vi "Smart Home Project.vi"() -> ()   [LabVIEW 2014]
doc: "This example demonstrates how to read one channel of digital input from a LINX device."
uses:
  <vilib>/MakerHub/LINX/Public/Peripherals/Digital/Digital Read 1 Chan.vi
  <vilib>/MakerHub/LINX/Public/Peripherals/Digital/Digital Write 1 Chan.vi
  <vilib>/MakerHub/LINX/Public/Peripherals/Analog/Analog Read 1 Chan.vi
  <vilib>/MakerHub/LINX/Public/Peripherals/PWM/PWM Set Duty Cycle 1 Chan.vi
  <vilib>/MakerHub/LINX/Public/Peripherals/Digital/Digital Read N Chans.vi
  <vilib>/MakerHub/LINX/Public/Peripherals/Digital/Digital Write N Chans.vi
  <vilib>/MakerHub/LINX/Public/Peripherals/Analog/Analog Read N Chans.vi
  <vilib>/MakerHub/LINX/Private/Local IO/LinxDigitalRead.vi
  <vilib>/MakerHub/LINX/Public/Utilities/Check Channel.vi
  <vilib>/MakerHub/LINX/Private/Local IO/LinxDigitalWrite.vi
  <vilib>/MakerHub/LINX/Private/Local IO/LinxAnalogRead.vi
  <vilib>/MakerHub/LINX/Public/Utilities/Open Serial.vi
  <vilib>/MakerHub/LINX/Public/Sensors/Motion/Servo/Servo Open One Channel.vi
  <vilib>/MakerHub/LINX/Private/Utilties/Generate Error.vi
  <vilib>/MakerHub/LINX/Public/Peripherals/PWM/PWM Set Duty Cycle N Chans.vi
  <vilib>/MakerHub/LINX/Public/Sensors/Motion/Servo/Servo Set Pulse Width One Channel.vi
  <vilib>/MakerHub/LINX/Public/Sensors/Motion/Servo/Servo Close One Channel.vi
  <vilib>/MakerHub/LINX/LMH-LINX.lvlib
  <vilib>/MakerHub/LINX/Public/Sensors/Motion/Servo/Servo.lvlib
panel:
  out "LDR Value":dbl
  out "Temp":dbl(slide) scale=0.0..50.0
  in  "Stop Button":bool
  out "TCR":bool
  out "Sound Sensor  Case":bool
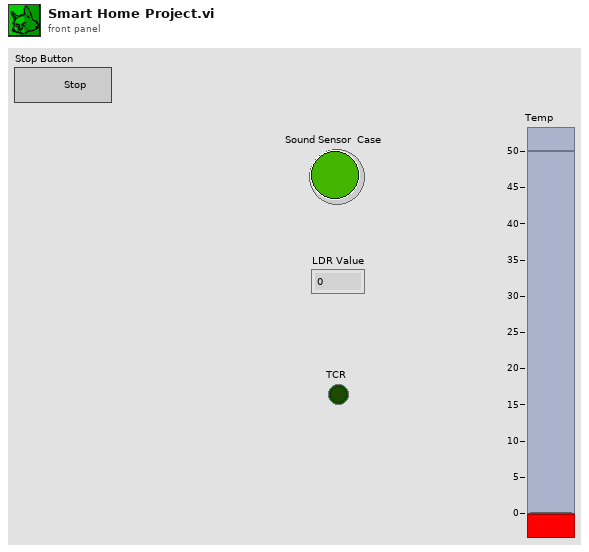
[diagram p1: front panel]
types:
  T1 = typedef "LMH-LINX.lvlib/LINX Ref.ctl" = cluster{"IO":T2, "Interface":T3, "LINX Device Config":T4}
  T2 = typedef "LMH-LINX.lvlib/Platform.ctl" = enum16{"Remote", "Local"}
  T3 = typedef "LMH-LINX.lvlib/Interface.ctl" = enum16{"Serial", "TCP"}
  T4 = typedef "LMH-LINX.lvlib/Device.lvlib/LINX Device Config.ctl" = cluster{"Interface":T3, "COM Port":refnum<visa-resource-name>, "TCP Configuration":T5, "Device Family":u8, "Device ID":u8, "Device Name":string, "TCP Ref":refnum<k5>, "Channels":T6}
  T5 = typedef "LMH-LINX.lvlib/Device.lvlib/TCP Config.ctl" = cluster{"IP Address":string, "Port":u16}
  T6 = typedef "LMH-LINX.lvlib/Channels.ctl" = cluster{"DI":u8[], "DO":u8[], "AI":u8[], "AO":u8[], "PWM":u8[], "QE":u8[], "UART":u8[], "I2C 2":u8[], "SPI":u8[], "CAN":u8[], "Servo":u8[], "AI Ref (V)":dbl, "AI Resolution (Bits)":u8, "AO Ref (V)":dbl, "AO Resolution (Bits)":u8}
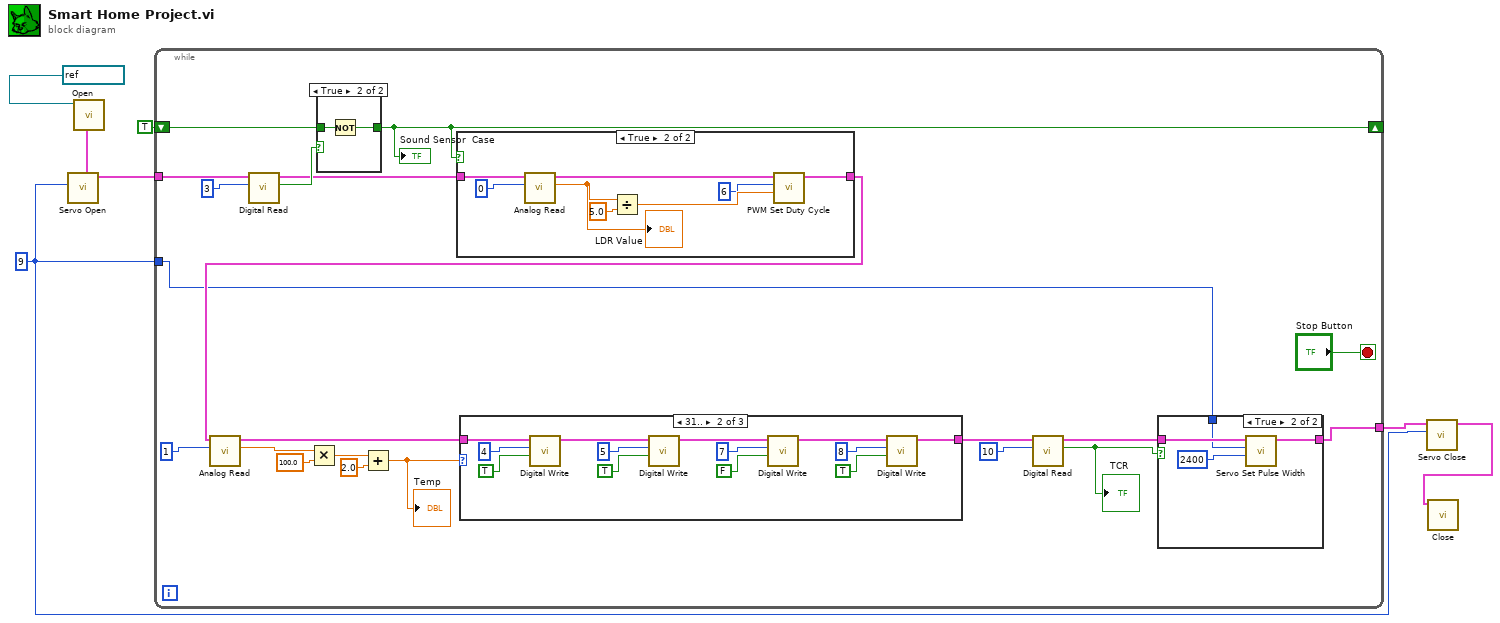
[diagram p0: block diagram]
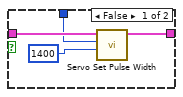
[diagram p2: hidden frame]
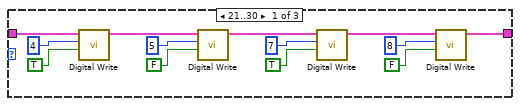
[diagram p3: hidden frame]
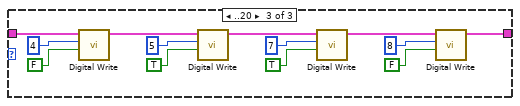
[diagram p4: hidden frame]
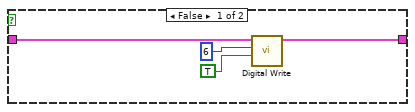
[diagram p5: hidden frame]
diagram:
  w1 = u8 9 ("Servo Channel")
  n1 = call-poly <vilib>:"Open.vi"("Serial Port"=refnum<visa-resource-name> "COM3") -> ("LINX Resource"=w4:T1)  [unwired: 8 in, 2 out]
  n2 = call-poly <vilib>:"Servo Open.vi"("Servo Channel"=w1, "LINX Resource"=w4) -> ("LINX Resource"=w5:T1)  [unwired: 8 in, 1 out]
  n3 = while {
    tunnel: w5 -> [w23]
    shift-right: [w26] -> _
    shift-left: TRUE -> [w28]
    tunnel: w1 -> [w9]
    tunnel: [w10] -> w3
    stop <- "Stop Button" stop-if-true
    n4 = call-poly <vilib>:"Digital Read.vi"("DI Channel"=u8 3, "LINX Resource"=w23) -> ("DI Value"=w27:bool, "LINX Resource"=w25:T1)  [unwired: 7 in, 1 out]
    n5 = case shown="True" w27 {
      tunnel: w28 -> [w88 w90]
      tunnel: [w88 w89] -> w26
      frame False {
      }
      frame True {
        n6 = Not(x=w90) -> (.not. x?=w89:bool)
      }
    }
    "Sound Sensor  Case" <- w26
    n7 = case shown="True" w26 {
      tunnel: w25 -> [w79 w87]
      tunnel: [w78 w81] -> w12
      frame False {
        n8 = call-poly <vilib>:"Digital Write.vi"("Output Value"=TRUE, "DO Channel"=u8 6, "LINX Resource"=w79) -> ("LINX Resource"=w78:T1)  [unwired: 7 in, 1 out]
      }
      frame True {
        n9 = call-poly <vilib>:"Analog Read.vi"("Analog Channel"=u8 0, "LINX Resource"=w87) -> ("Voltage"=w80:dbl, "LINX Resource"=w82:T1)  [unwired: 6 in, 2 out]
        "LDR Value" <- w80
        n10 = Divide(x=w80, y=5.0) -> (x/y=w86:dbl)
        n11 = call-poly <vilib>:"PWM Set Duty Cycle.vi"("Duty Cycle (0-1)"=w86, "PWM Channel"=u8 6, "LINX Resource"=w82) -> ("LINX Resource"=w81:T1)  [unwired: 7 in, 1 out]
      }
    }
    n12 = call-poly <vilib>:"Analog Read.vi"("Analog Channel"=u8 1, "LINX Resource"=w12) -> ("Voltage"=w20:dbl, "LINX Resource"=w17:T1)  [unwired: 6 in, 2 out]
    n13 = Multiply(x=w20, y=100.0) -> (x*y=w22:dbl)
    n14 = Add(x=w22, y=2.0) -> (x+y=w8:dbl)
    "Temp" <- w8
    n15 = case shown="31.." w8 {
      tunnel: w17 -> [w49 w58 w67]
      tunnel: [w37 w50 w63] -> w16
      frame 21..30 {
        n16 = call-poly <vilib>:"Digital Write.vi"("Output Value"=TRUE, "DO Channel"=u8 4, "LINX Resource"=w49) -> ("LINX Resource"=w48:T1)  [unwired: 7 in, 1 out]
        n17 = call-poly <vilib>:"Digital Write.vi"("Output Value"=FALSE, "DO Channel"=u8 5, "LINX Resource"=w48) -> ("LINX Resource"=w47:T1)  [unwired: 7 in, 1 out]
        n18 = call-poly <vilib>:"Digital Write.vi"("Output Value"=TRUE, "DO Channel"=u8 7, "LINX Resource"=w47) -> ("LINX Resource"=w46:T1)  [unwired: 7 in, 1 out]
        n19 = call-poly <vilib>:"Digital Write.vi"("Output Value"=FALSE, "DO Channel"=u8 8, "LINX Resource"=w46) -> ("LINX Resource"=w37:T1)  [unwired: 7 in, 1 out]
      }
      frame 31.. {
        n20 = call-poly <vilib>:"Digital Write.vi"("Output Value"=TRUE, "DO Channel"=u8 4, "LINX Resource"=w58) -> ("LINX Resource"=w57:T1)  [unwired: 7 in, 1 out]
        n21 = call-poly <vilib>:"Digital Write.vi"("Output Value"=TRUE, "DO Channel"=u8 5, "LINX Resource"=w57) -> ("LINX Resource"=w56:T1)  [unwired: 7 in, 1 out]
        n22 = call-poly <vilib>:"Digital Write.vi"("Output Value"=FALSE, "DO Channel"=u8 7, "LINX Resource"=w56) -> ("LINX Resource"=w55:T1)  [unwired: 7 in, 1 out]
        n23 = call-poly <vilib>:"Digital Write.vi"("Output Value"=TRUE, "DO Channel"=u8 8, "LINX Resource"=w55) -> ("LINX Resource"=w50:T1)  [unwired: 7 in, 1 out]
      }
      frame ..20 {
        n24 = call-poly <vilib>:"Digital Write.vi"("Output Value"=FALSE, "DO Channel"=u8 4, "LINX Resource"=w67) -> ("LINX Resource"=w66:T1)  [unwired: 7 in, 1 out]
        n25 = call-poly <vilib>:"Digital Write.vi"("Output Value"=TRUE, "DO Channel"=u8 5, "LINX Resource"=w66) -> ("LINX Resource"=w65:T1)  [unwired: 7 in, 1 out]
        n26 = call-poly <vilib>:"Digital Write.vi"("Output Value"=TRUE, "DO Channel"=u8 7, "LINX Resource"=w65) -> ("LINX Resource"=w64:T1)  [unwired: 7 in, 1 out]
        n27 = call-poly <vilib>:"Digital Write.vi"("Output Value"=FALSE, "DO Channel"=u8 8, "LINX Resource"=w64) -> ("LINX Resource"=w63:T1)  [unwired: 7 in, 1 out]
      }
    }
    n28 = call-poly <vilib>:"Digital Read.vi"("DI Channel"=u8 10, "LINX Resource"=w16) -> ("DI Value"=w13:bool, "LINX Resource"=w15:T1)  [unwired: 7 in, 1 out]
    "TCR" <- w13
    n29 = case shown="True" w13 {
      tunnel: w15 -> [w30 w36]
      tunnel: [w32 w34] -> w10
      tunnel: w9 -> [w29 w33]
      frame False {
        n30 = call-poly <vilib>:"Servo Set Pulse Width.vi"("Pulse Width (uS)"=u16 1400, "Servo Channel"=w29, "LINX Resource"=w30) -> ("LINX Resource"=w32:T1)  [unwired: 7 in, 1 out]
      }
      frame True {
        n31 = call-poly <vilib>:"Servo Set Pulse Width.vi"("Pulse Width (uS)"=u16 2400, "Servo Channel"=w33, "LINX Resource"=w36) -> ("LINX Resource"=w34:T1)  [unwired: 7 in, 1 out]
      }
    }
  }
  n32 = call-poly <vilib>:"Servo Close.vi"("Servo Channel"=w1, "LINX Resource"=w3) -> ("LINX Resource"=w2:T1)  [unwired: 8 in, 1 out]
  n33 = call <vilib>:"Close.vi"("LINX Resource"=w2) -> ()  [unwired: 10 in, 1 out]
